vi "Self Messaging.vi"() -> (3 "Pass?":bool)   [LabVIEW 2023]
uses:
  <vilib>/ActorFramework/LastAck/Last Ack.lvclass
  TestActor2/TestActor2.lvclass
  C:/Program Files/National Instruments/LabVIEW 2024/vi.lib/ActorFramework/Actor/Actor.lvclass
  <vilib>/ActorFramework/Message Queue/Message Queue.lvclass/Message Queue.ctl
  Increment2 Msg/Increment2 Msg.lvclass/Increment2 Msg.ctl
  <vilib>/ActorFramework/Message Enqueuer/Message Enqueuer.lvclass/Message Enqueuer.ctl
  <vilib>/ActorFramework/Message Dequeuer/Message Dequeuer.lvclass/Message Dequeuer.ctl
  <vilib>/ActorFramework/LastAck/Last Ack.lvclass/Last Ack.ctl
  TestActor2/TestActor2.lvclass/TestActor2.ctl
  <vilib>/ActorFramework/Message Enqueuer/Enqueue.vi
  Increment2 Msg/Increment2 Msg.lvclass
  C:/Program Files/National Instruments/LabVIEW 2024/vi.lib/ActorFramework/Message/Message.lvclass
  <vilib>/ActorFramework/Message Priority Queue/Priority Dequeue.vi
  <vilib>/ActorFramework/Message Priority Queue/Priority Enqueue.vi
  <vilib>/ActorFramework/Actor/Actor.lvclass
  <vilib>/ActorFramework/Message Queue/Message Queue.lvclass
  <vilib>/ActorFramework/Message Dequeuer/Message Dequeuer.lvclass
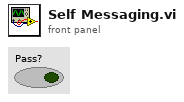
[diagram p1: front panel]
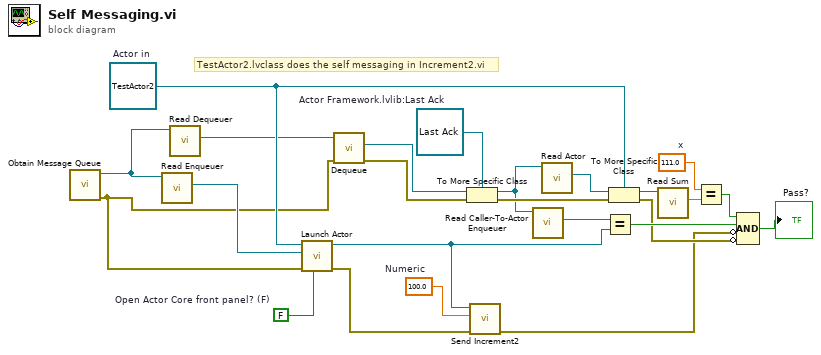
[diagram p0: block diagram]
diagram:
  w12 = refnum<class "TestActor2.lvclass"> refnum  # Actor in
  w13 = FALSE  # Open Actor Core front panel? (F)
  w21 = 111.0  # x
  w24 = refnum<class "Last Ack.lvclass"> refnum  # Actor Framework.lvlib:Last Ack
  w16 = 100.0  # Numeric
  # "TestActor2.lvclass does the self messaging in Increment2.vi"
  n1 = call <vilib>:"Obtain Message Queue.vi"() -> ("error out"=w4:errorcluster, "Message Queue"=w8:refnum<class "Message Queue.lvclass">)  [unwired: 10 in]
  n2 = call <vilib>:"Read Enqueuer.vi"("Message Queue"=w8) -> ("Message Enqueuer"=w7:refnum<class "Message Enqueuer.lvclass">)  [unwired: 10 in]
  n3 = call <vilib>:"Read Dequeuer.vi"("Message Queue"=w8) -> ("Message Dequeuer"=w6:refnum<class "Message Dequeuer.lvclass">)  [unwired: 10 in]
  n4 = call <vilib>:"Launch Actor.vi"("Open Actor Core front panel? (F)"=w13, "error in (no error)"=w4, "Actor-to-Caller Enqueuer"=w7, "Actor"=w12) -> ("error out"=w14:errorcluster, "Caller-To-Actor Enqueuer"=w15:refnum<class "Message Enqueuer.lvclass">)  [unwired: 6 in]
  n5 = call <vilib>:"Dequeue.vi"("error in (no error)"=w4, "Message Dequeuer in"=w6) -> ("error out"=w3:errorcluster, "Message"=w5:refnum<class "Message.lvclass">)  [unwired: 5 in, 3 out]
  n6 = To More Specific Class(target class=w24, reference=w5, error in=w3) -> (specific class reference=w2:refnum<class "Last Ack.lvclass">, error out=w23:errorcluster)
  n7 = call "Send Increment2.vi"("error in (no error)"=w14, "Numeric"=w16, "Message Enqueuer"=w15) -> ("error out"=w9:errorcluster)  [unwired: 8 in]
  n8 = call <vilib>:"Read Caller-To-Actor Enqueuer.vi"("Last Ack"=w2) -> ("Caller-to-Actor Enqueuer"=w1:refnum<class "Message Enqueuer.lvclass">)  [unwired: 10 in]
  n9 = call <vilib>:"Read Actor.vi"("Last Ack"=w2) -> ("Actor"=w22:refnum<class "Actor.lvclass">)  [unwired: 10 in]
  n10 = Equal?(x=w1, y=w15) -> (x = y?=w19:bool)
  n11 = To More Specific Class(target class=w12, reference=w22, error in=w23) -> (specific class reference=w11:refnum<class "TestActor2.lvclass">, error out=w17:errorcluster)
  n12 = call "Read Sum.vi"("TestActor in"=w11) -> ("Sum"=w10:dbl)  [unwired: 9 in, 1 out]
  n13 = Equal?(x=w21, y=w10) -> (x = y?=w20:bool)
  n14 = Compound Arithmetic op=AND(w20, w19, invert w9, invert w17) -> (→"Pass?":bool)
